vi "kdbTestCRUD.vi"() -> ()   [LabVIEW 2020, in "ORM_Examples.lvlib"]
uses:
  ORM_Examples.lvlib
  Vehicle/Vehicle.lvclass
  VehicleMap/VehicleMap.lvclass
  C:/Program Files/National Instruments/LabVIEW 2020/vi.lib/Viviota/shared/ORM.lvlibp/ORM/TypeMap/TypeMap.lvclass
  <vilib>/Viviota/shared/ORM_DBC_Kdb.lvlibp/DBC.lvclass
  C:/Program Files/National Instruments/LabVIEW 2020/vi.lib/Viviota/shared/ORM.lvlibp/ORM/DbConnection/DbConnection.lvclass
  <vilib>/Viviota/shared/ORM_ADONet.lvlibp/ADOMapper/ADOMapper.lvclass
  C:/Program Files/National Instruments/LabVIEW 2020/vi.lib/Viviota/shared/ORM.lvlibp/ORM/SqlMapper/SqlMapper.lvclass
  Vehicle/Vehicle.lvclass/Vehicle.ctl
  Vehicle/Write Make.vi
  Vehicle/Write Model.vi
  Vehicle/Write Year.vi
  Vehicle/Write VehicleID.vi
  7921b66d-6ce7-4af3-949e-ef797308c048.vi
  8fb8b2d8-1472-417a-b089-fe21007d0a1a.vi
  ed13316f-6b3d-4b66-9e50-d6175327a74a.vi
  c2d1a64a-a3d4-455d-b464-a513ccf986a2.vi
  d40dc63b-9994-4387-bfea-9e10b8447491.vi
  Vehicle/Read Make.vi
  Vehicle/Read Model.vi
  Vehicle/Read Year.vi
  Vehicle/Read VehicleID.vi
  7921b66d-6ce7-4af3-949e-ef797308c048.vi/35b31214-e0d6-4ae0-b34c-13eba9df70db.vi
  7921b66d-6ce7-4af3-949e-ef797308c048.vi/2e8f1eab-5a58-47e6-9224-d0a2895e31fd.vi
  8fb8b2d8-1472-417a-b089-fe21007d0a1a.vi/ce8babb2-619c-4b95-b634-e027cd54a13e.vi
  8fb8b2d8-1472-417a-b089-fe21007d0a1a.vi/383c36e0-7191-4c70-923d-4cc1411f3794.vi
  8fb8b2d8-1472-417a-b089-fe21007d0a1a.vi/dcffdf9a-60b2-440f-af14-9d618c05381d.vi
  ed13316f-6b3d-4b66-9e50-d6175327a74a.vi/bf74eca6-e633-4dc5-891a-edef426d4fd9.vi
  c2d1a64a-a3d4-455d-b464-a513ccf986a2.vi/93c2cd5d-a53a-4cc2-b8c3-9c3eef6598b6.vi
  d40dc63b-9994-4387-bfea-9e10b8447491.vi/a9ccc3c9-891a-4d80-8d4f-837bdef88ccd.vi
  d40dc63b-9994-4387-bfea-9e10b8447491.vi/8216614f-f413-45b3-8111-14f8d0271ea5.vi
  d40dc63b-9994-4387-bfea-9e10b8447491.vi/fc6a5c23-d21f-4d2c-895e-66da96fa9491.vi
  d40dc63b-9994-4387-bfea-9e10b8447491.vi/fc6a5c23-d21f-4d2c-895e-66da96fa9491.vi/9d007ba8-e96f-4737-8d8a-6b46cf7f5c4a.vi
  d40dc63b-9994-4387-bfea-9e10b8447491.vi/fc6a5c23-d21f-4d2c-895e-66da96fa9491.vi/050765a8-e5d4-4415-b637-62775228e838.vi
  <vilib>/Viviota/shared/ORM.lvlibp/ORM/SqlMapper/Write DbConnection.vi
  <vilib>/Utility/error.llb/Error Cluster From Error Code.vi
  <vilib>/Viviota/shared/ORM.lvlibp/ORM/TypeMap/Read TypeMap.vi
  <vilib>/Viviota/shared/ORM.lvlibp/ORM/SqlMapper/End Transaction.vi
  <vilib>/Viviota/shared/ORM.lvlibp/ORM/TypeMap/Where.vi
  <vilib>/Viviota/shared/ORM.lvlibp/ORM/Query Result/Next.vi
  <vilib>/Viviota/shared/ORM.lvlibp/ORM/TypeMap/ToLabVIEW_Wrap.vi
  <vilib>/Viviota/shared/ORM.lvlibp/ORM/TypeMap/TypeMap.lvclass
  <vilib>/Viviota/shared/ORM.lvlibp/ORM/Query Result/Query Result.lvclass
panel:
  in  "Array":string[](array[string])
  out "output cluster":T1(array[cluster])
  out "error out 2":errorcluster
  in  "Port":u16=5000
  in  "Enum":T2(ring)
  out "error out":errorcluster
  out "affectedRows":i32
  in  "VehicleCluster":T3={"Make"="Honda", "Model"="Civic", "Year"=2018, "ID"=2018}
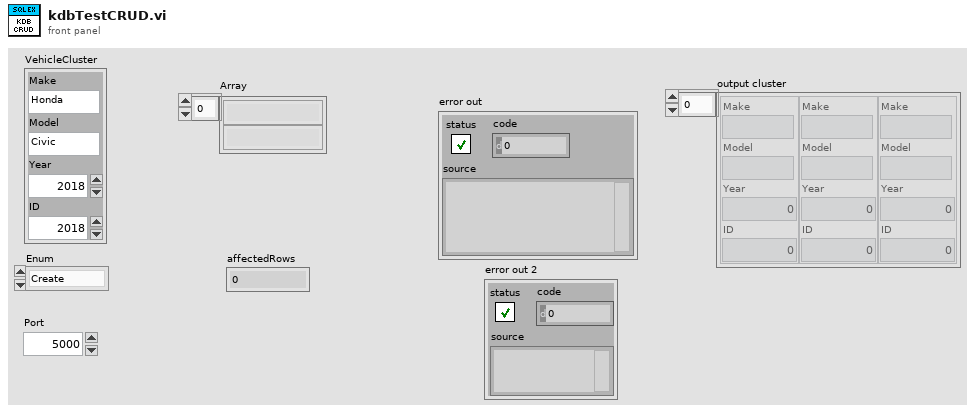
[diagram p1: front panel]
types:
  T1 = cluster{"Make":string, "Model":string, "Year":i32, "ID":i32}[]
  T2 = enum16{"Create", "Read", "Update", "Destroy", "ReadAll"}
  T3 = cluster{"Make":string, "Model":string, "Year":i32, "ID":i32}
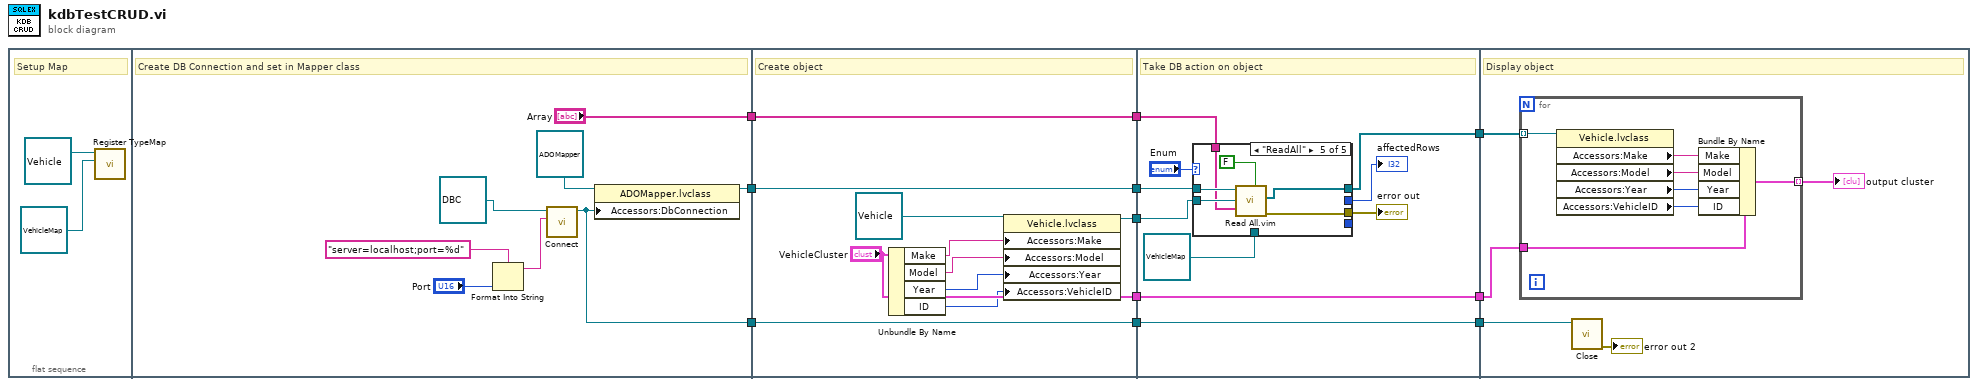
[diagram p0: block diagram]
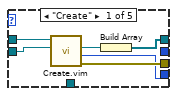
[diagram p2: hidden frame]
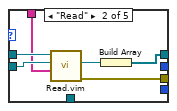
[diagram p3: hidden frame]
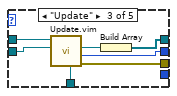
[diagram p4: hidden frame]
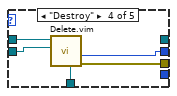
[diagram p5: hidden frame]
diagram:
  n1 = flat-sequence {
    tunnel: [w21] -> w11
    tunnel: [w15] -> w3
    tunnel: ["Array"] -> w1
    tunnel: w11 -> [w30]
    tunnel: ["VehicleCluster"] -> w10
    tunnel: [w31] -> w9
    tunnel: [w30] -> w8
    tunnel: [w24] -> w4
    tunnel: w3 -> [w24]
    tunnel: [w22] -> w2
    tunnel: w1 -> [w22]
    tunnel: w10 -> [w37]
    tunnel: w9 -> [w39]
    tunnel: w8 -> [w38]
    tunnel: [w37] -> w7
    tunnel: [w36] -> w6
    tunnel: [w33] -> w5
    tunnel: w4 -> [w33]
    tunnel: w2 -> [w32]
    tunnel: w7 -> [w72]
    tunnel: w6 -> [w76]
    tunnel: w5 -> [w75]
    frame #0 {
      # "Setup Map"
      n2 = call <vilib>:"Register TypeMap.vi"("TypeMap in"=refnum<class "VehicleMap.lvclass"> refnum ("VehicleMap.lvclass"), "object in"=refnum<class "Vehicle.lvclass"> refnum ("Vehicle.lvclass")) -> ()  [unwired: 7 in, 3 out]
    }
    frame #1 {
      # "Create DB Connection and set in Mapper class"
      n3 = Format Into String(format string="server=localhost;port=%d" ("connectionStringName"), "Port") -> (resulting string=w17:string)  [unwired: 2 in, 1 out]
      n4 = call-dynamic "Connect.vi"("Connection String"=w17, "SqliteConnection in"=refnum<class "DBC.lvclass"> refnum ("KDBConnection.lvclass")) -> ("SqliteConnection out"=w15:refnum<class "DBC.lvclass">)  [unwired: 8 in, 1 out]
      n5 = property class="ADOMapper.lvclass"(reference=refnum<class "ADOMapper.lvclass"> refnum ("ADONet.lvlib:ADOMapper.lvclass"), "Accessors:DbConnection"=w15) -> (reference out=w21:refnum<class "ADOMapper.lvclass">)  [unwired: 1 in, 1 out]
    }
    frame #2 {
      # "Create object"
      n6 = Unbundle By Name("VehicleCluster") -> ("Make"=w28:string, "Model"=w27:string, "Year"=w26:i32, "ID"=w23:i32)
      n7 = property class="Vehicle.lvclass"(reference=refnum<class "Vehicle.lvclass"> refnum ("Vehicle.lvclass"), "Accessors:Make"=w28, "Accessors:Model"=w27, "Accessors:Year"=w26, "Accessors:VehicleID"=w23) -> (reference out=w31:refnum<class "Vehicle.lvclass">)  [unwired: 1 in, 1 out]
    }
    frame #3 {
      # "Take DB action on object"
      n8 = case shown="\"ReadAll\"" "Enum" {
        tunnel: w39 -> [w46 w52 w56 w64 w70]
        tunnel: w38 -> [w47 w53 w60 w65 w71]
        tunnel: [w42 w49 w54 _ w68] -> w36
        tunnel: [w44 w50 w57 w63 w67] -> w41
        tunnel: [_ _ w58 w62 _] -> w35
        tunnel: refnum<class "VehicleMap.lvclass"> refnum ("VehicleMap.lvclass") -> [_ _ w55 w61 _]
        tunnel: [w43 _ _ _ _] -> _
        tunnel: w32 -> [_ w48 _ _ w66]
        frame "Create" {
          n9 = call "Create.vim"("object in"=w46, "SqlMapper in"=w47) -> ("error out"=w44:errorcluster, "id"=w43:i32, "object out"=w45:refnum<class "Vehicle.lvclass">)  [unwired: 6 in, 1 out]
          n10 = Build Array(w45) -> (w42:refnum<class "Vehicle.lvclass">[])
        }
        frame "Read" {
          n11 = call "Read.vim"("Where"=w48, "object in"=w52, "SqlMapper in"=w53) -> ("error out"=w50:errorcluster, "object out"=w51:refnum<class "Vehicle.lvclass">)  [unwired: 5 in, 2 out]
          n12 = Build Array(w51) -> (w49:refnum<class "Vehicle.lvclass">[])
        }
        frame "Update" {
          n13 = call "Update.vim"("TypeMap in"=w55, "object in"=w56, "SqlMapper in"=w60) -> ("error out"=w57:errorcluster, "affectedRows"=w58:i32, "object out"=w59:refnum<class "Vehicle.lvclass">)  [unwired: 5 in, 1 out]
          n14 = Build Array(w59) -> (w54:refnum<class "Vehicle.lvclass">[])
        }
        frame "Destroy" {
          n15 = call "Delete.vim"("TypeMap in"=w61, "object in"=w64, "SqlMapper in"=w65) -> ("error out"=w63:errorcluster, "affectedRows"=w62:i32)  [unwired: 6 in, 1 out]
        }
        frame "ReadAll" {
          n16 = call "Read All.vim"("Select All"=FALSE ("Select *"), "WHERE"=w66, "Object"=w70, "SqlMapper in"=w71) -> ("error out"=w67:errorcluster, "Query Results"=w68:refnum<class "Vehicle.lvclass">[])  [unwired: 5 in, 1 out]
        }
      }
      "error out" <- w41
      "affectedRows" <- w35
    }
    frame #4 {
      # "Display object"
      n17 = for {
        tunnel: w76 -> [w81] mode=indexing
        tunnel: [w78] -> w73 mode=indexing
        tunnel: w72 -> [w77]
        n18 = property class="Vehicle.lvclass"(reference=w81) -> ("Accessors:Make"=w83:string, "Accessors:Model"=w82:string, "Accessors:Year"=w80:i32, "Accessors:VehicleID"=w79:i32)  [unwired: 1 in, 2 out]
        n19 = Bundle By Name(cluster=w77, "Make"=w83, "Model"=w82, "Year"=w80, "ID"=w79) -> (w78:T3)
      }
      "output cluster" <- w73
      n20 = call-dynamic "Close.vi"("dbcDotNet in"=w75) -> ("error out"=→"error out 2":errorcluster)  [unwired: 10 in]
    }
  }
